vi "fisiere_v0.vi"() -> ()   [LabVIEW 2009]
panel:
  out "String":string
  in  "Selectati calea si fisierul":path=path "E:/Projects/Lab_view/Vi/fisiere/country-capital.txt"
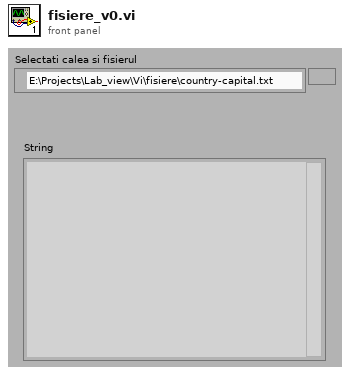
[diagram p1: front panel]
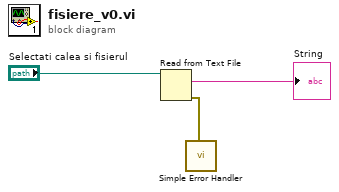
[diagram p0: block diagram]
diagram:
  n1 = Read from Text File(file (use dialog)="Selectati calea si fisierul") -> (text=→"String":string, error out=w2:errorcluster)  [unwired: 3 in, 2 out]
  n2 = call <vilib>:"Simple Error Handler.vi"("error in (no error)"=w2) -> ()  [unwired: 4 in, 5 out]
